vi "Demo.vi"() -> ()   [LabVIEW 2014, in "XGaussfitGraph.lvlib"]
uses:
  XGaussfitGraph.lvlib
  XGaussfitGraph.xctl
  <vilib>/Analysis/NI_AALBase.lvlib
panel:
  out "Waveform Graph":dbl[](graph)
  out "Gaussian noise pattern":dbl[](array[numeric])
  out "XGaussfitGraph":dbl[](xcontrol)
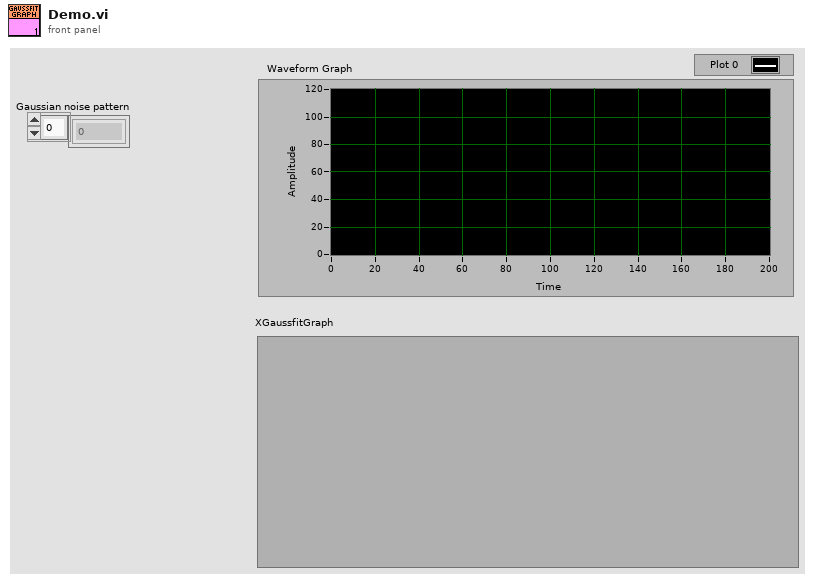
[diagram p1: front panel]
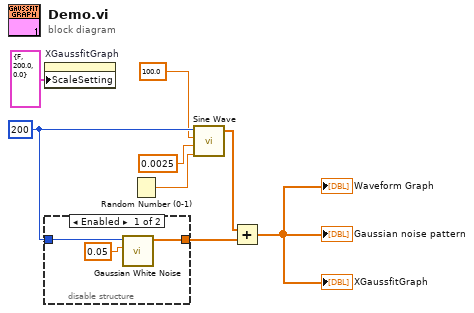
[diagram p0: block diagram]
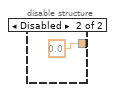
[diagram p2: hidden frame]
diagram:
  w7 = 200 ("Numeric")
  n1 = property on="XGaussfitGraph" class="XGaussfitGraph (strict)"("ScaleSetting"=cluster{"auto?":bool, "max":dbl, "min":dbl} {"auto?"=FALSE, "max"=200.0, "min"=0.0}) -> ()  [unwired: 2 in, 2 out]
  n2 = disable-structure shown="Enabled" {
    disable-tunnel: [w11 0.0] -> w8
    disable-tunnel: w7 -> [w9 _]
    frame Enabled {
      n3 = call <vilib>:"Gaussian White Noise.vi"("standard deviation"=0.05, "samples"=w9) -> ("Gaussian noise pattern"=w11:dbl[])  [unwired: 8 in, 1 out]
    }
    frame Disabled {
    }
  }
  n4 = Random Number (0-1)() -> (number: 0 to 1=w3:dbl)
  n5 = call <vilib>:"Sine Wave.vi"("samples"=w7, "amplitude"=100.0, "frequency"=0.0025, "phase in"=w3) -> ("sine wave"=w6:dbl[])  [unwired: 1 in, 2 out]
  n6 = Add(x=w6, y=w8) -> (x+y=→"XGaussfitGraph" →"Gaussian noise pattern" →"Waveform Graph":dbl[])
